vi "DFT.vi"(0 "dt":dbl=0.001, 1 "Input Y":dbl[](array[numeric]), 3 "Input X":dbl[](array[numeric]), 5 "df":dbl=1.0, 9 "fmin":dbl, 11 "fmax":dbl=500.0, 12 "Windowing":T3=enum."Sine", 13 "Autocorrelation before DFT":T1, 14 "Mean shifting":T2) -> (4 "Pwr out":dbl[](array[numeric]), 6 "fnyq.":dbl, 8 "Input to DFT":dbl[](graph), 10 "Actual fmin":dbl, 15 "Actual fmax":dbl)   [LabVIEW 2011]
uses:
  Windowing_list.ctl
  Mean_shift_list.ctl
  Autocorrelation_list.ctl
  <vilib>/Analysis/4window.llb/Cosine Tapered Window (DBL).vi
  <vilib>/Analysis/4window.llb/Triangle Window (DBL).vi
  <vilib>/Analysis/4window.llb/Exact Blackman Window (DBL).vi
  <vilib>/Analysis/4window.llb/Flat Top Window (DBL).vi
  <vilib>/Analysis/4window.llb/Hamming Window (DBL).vi
  <vilib>/Analysis/4window.llb/Hanning Window (DBL).vi
  <vilib>/Analysis/4window.llb/Blackman Window (DBL).vi
  <vilib>/Analysis/4window.llb/Blackman-Harris Window (DBL).vi
  <vilib>/Analysis/2dsp.llb/1D Auto Correlation (DBL).vi
  <vilib>/Analysis/NI_AALBase.lvlib
  <vilib>/Analysis/NI_AALPro.lvlib
panel:
  out "Variance Density Spectrum":cluster{"fmin":dbl, "df":dbl, dbl[]}(graph)
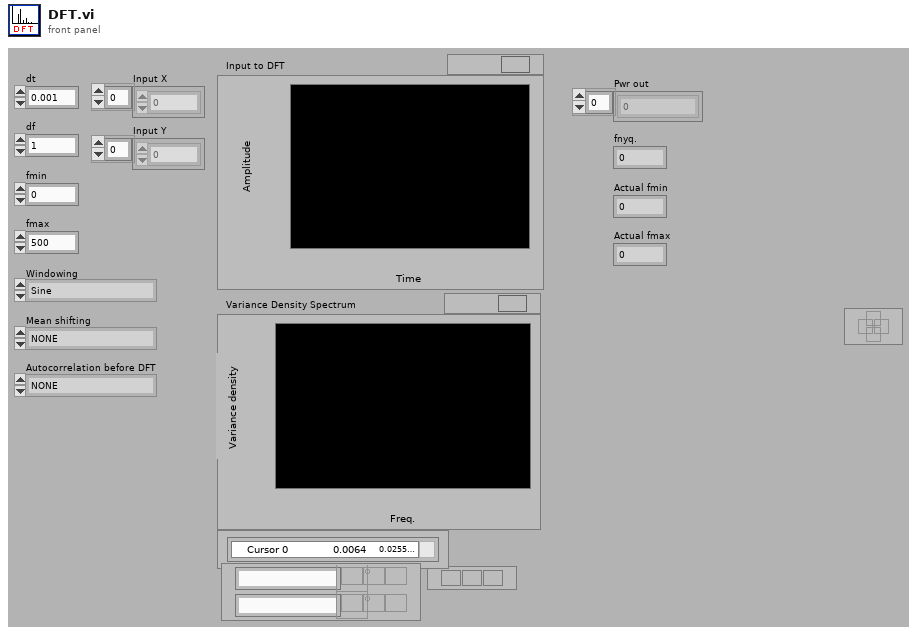
[diagram p1: front panel]
types:
  T1 = typedef "Autocorrelation_list.ctl" = enum16{"NONE", "Biased", "Un-biased"}
  T2 = typedef "Mean_shift_list.ctl" = enum16{"NONE", "Eliminate DC only", "Eliminate all linear trends"}
  T3 = typedef "Windowing_list.ctl" = enum16{"NONE", "Blackman", "Blackman Harris", "Cosine Taper", "Exact Blackman", "Flat Top", "Hamming", "Hanning", "Sine", "Triangle"}
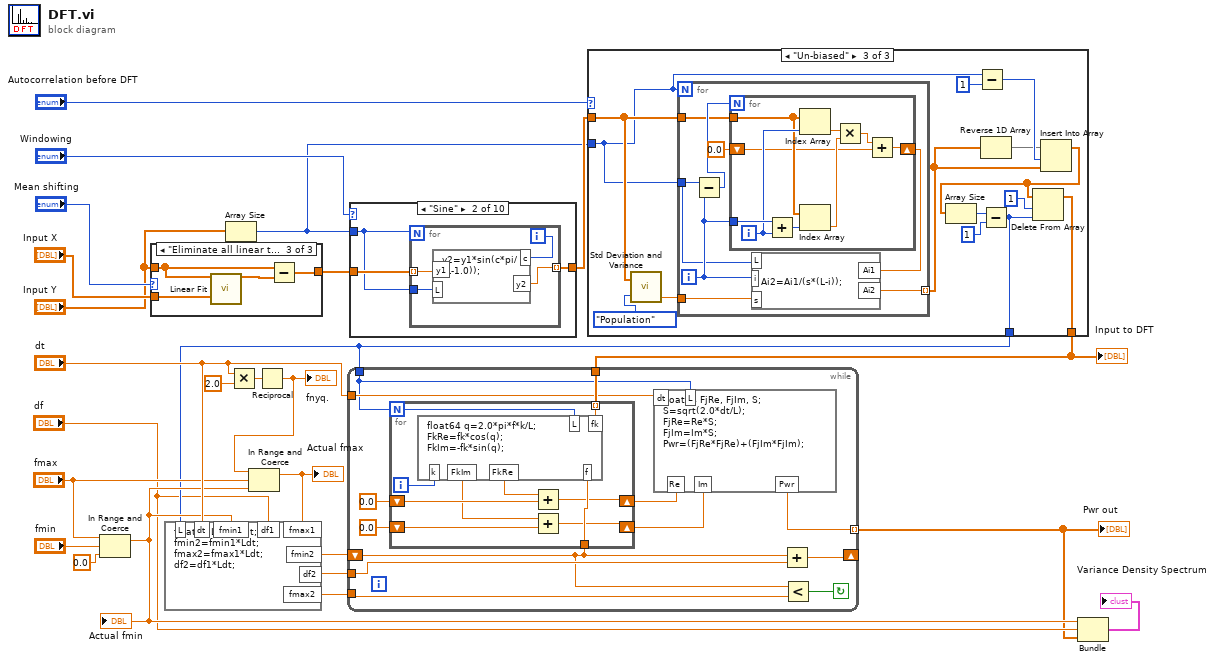
[diagram p0: block diagram]
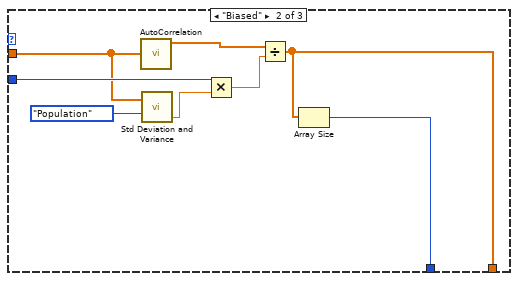
[diagram p3: hidden frame]
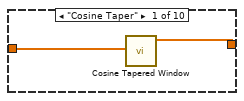
[diagram p4: hidden frame]
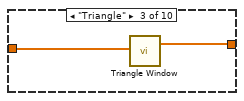
[diagram p5: hidden frame]
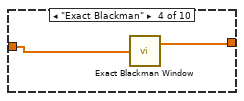
[diagram p6: hidden frame]
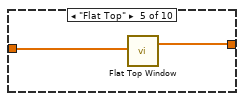
[diagram p7: hidden frame]
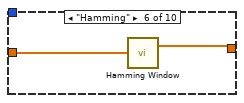
[diagram p8: hidden frame]
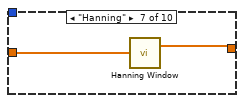
[diagram p9: hidden frame]
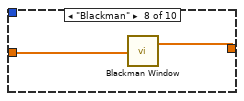
[diagram p10: hidden frame]
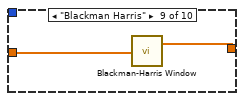
[diagram p11: hidden frame]
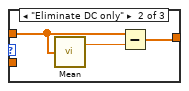
[diagram p14: hidden frame]
diagram:
  n1 = In Range and Coerce(upper limit="fmax", x="fmin", lower limit=0.0) -> (coerced(x)=w13:dbl)  [unwired: 1 out]
  "Actual fmin" <- w13
  n2 = case shown="\"Eliminate all linear trends\"" "Mean shifting" {
    tunnel: "Input Y" -> [w26 w27 w31]
    tunnel: [w26 w29 w30] -> w9
    tunnel: "Input X" -> [_ _ w33]
    frame "NONE" {
    }
    frame "Eliminate DC only" {
      n3 = call <vilib>:"Mean.vi"("X"=w27) -> ("mean"=w28:dbl)  [unwired: 1 out]
      n4 = Subtract(x=w27, y=w28) -> (x-y=w29:dbl[])
    }
    frame "Eliminate all linear trends" {
      n5 = call <vilib>:"Linear Fit.vi"("Y"=w31, "X"=w33) -> ("Best Linear Fit"=w32:dbl[])  [unwired: 9 in, 4 out]
      n6 = Subtract(x=w31, y=w32) -> (x-y=w30:dbl[])
    }
  }
  n7 = Array Size(array="Input Y") -> (size(s)=w4:i32)
  n8 = Multiply(x="dt", y=2.0) -> (x*y=w24:dbl)
  n9 = Reciprocal(x=w24) -> (1/x=w18:dbl)
  "fnyq." <- w18
  n10 = In Range and Coerce(upper limit=w18, x="fmax", lower limit=w13) -> (coerced(x)=w17:dbl)  [unwired: 1 out]
  "Actual fmax" <- w17
  n11 = case shown="\"Sine\"" "Windowing" {
    tunnel: w9 -> [w35 w37 w44 w46 w48 w50 w52 w54 w56 w57]
    tunnel: [w34 w38 w43 w45 w47 w49 w51 w53 w55 w57] -> w7
    tunnel: w4 -> [_ w36 _ _ _ _ _ _ _ _]
    frame "Cosine Taper" {
      n12 = call-poly <vilib>:"Cosine Tapered Window.vi"("X"=w35) -> ("Windowed X"=w34:dbl[])  [unwired: 9 in, 1 out]
    }
    frame "Sine" {
      n13 = for {
        N: w36 -> [_]
        tunnel: w37 -> [w42] mode=indexing
        tunnel: w36 -> [w41]
        tunnel: [w40] -> w38 mode=indexing
        i -> [w39]
        n14 = formula code="y2=y1*sin(c*pi/(L-1.0));"("y1"=w42, "L"=w41, "c"=w39) -> ("y2"=w40:dbl)
      }
    }
    frame "Triangle" {
      n15 = call-poly <vilib>:"Triangle Window.vi"("X"=w44) -> ("Windowed X"=w43:dbl[])  [unwired: 1 out]
    }
    frame "Exact Blackman" {
      n16 = call-poly <vilib>:"Exact Blackman Window.vi"("X"=w46) -> ("Windowed X"=w45:dbl[])  [unwired: 1 out]
    }
    frame "Flat Top" {
      n17 = call-poly <vilib>:"Flat Top Window.vi"("X"=w48) -> ("Windowed X"=w47:dbl[])  [unwired: 1 out]
    }
    frame "Hamming" {
      n18 = call-poly <vilib>:"Hamming Window.vi"("X"=w50) -> ("Windowed X"=w49:dbl[])  [unwired: 1 out]
    }
    frame "Hanning" {
      n19 = call-poly <vilib>:"Hanning Window.vi"("X"=w52) -> ("Windowed X"=w51:dbl[])  [unwired: 1 out]
    }
    frame "Blackman" {
      n20 = call-poly <vilib>:"Blackman Window.vi"("X"=w54) -> ("Windowed X"=w53:dbl[])  [unwired: 1 out]
    }
    frame "Blackman Harris" {
      n21 = call-poly <vilib>:"Blackman-Harris Window.vi"("X"=w56) -> ("Windowed X"=w55:dbl[])  [unwired: 1 out]
    }
    frame "NONE" {
    }
  }
  n22 = case shown="\"Un-biased\"" "Autocorrelation before DFT" {
    tunnel: w7 -> [w59 w61 w81]
    tunnel: [w58 w67 w68] -> w6
    tunnel: [w59 w65 w72] -> w1
    tunnel: w4 -> [w58 w64 w77]
    frame "NONE" {
    }
    frame "Biased" {
      n23 = call-poly <vilib>:"AutoCorrelation.vi"("X"=w61) -> ("Rxx"=w66:dbl[])  [unwired: 9 in, 1 out]
      n24 = call <vilib>:"Std Deviation and Variance.vi"("X"=w61, "Weighting (Sample)"=enum16{"Sample", "Population"}."Population") -> ("variance"=w62:dbl)  [unwired: 2 out]
      n25 = Multiply(x=w64, y=w62) -> (x*y=w63:dbl)
      n26 = Divide(x=w66, y=w63) -> (x/y=w65:dbl[])
      n27 = Array Size(array=w65) -> (size(s)=w67:i32)
    }
    frame "Un-biased" {
      n28 = call <vilib>:"Std Deviation and Variance.vi"("X"=w81, "Weighting (Sample)"=enum16{"Sample", "Population"}."Population") -> ("variance"=w79:dbl)  [unwired: 2 out]
      n29 = for {
        N: w77 -> [_]
        tunnel: w77 -> [w82]
        tunnel: w81 -> [w85]
        tunnel: w79 -> [w88]
        tunnel: [w86] -> w74 mode=indexing
        i -> [w87]
        n30 = Subtract(x=w82, y=w87) -> (x-y=w89:i32)
        n31 = for {
          N: w89 -> [_]
          tunnel: w87 -> [w96]
          tunnel: w85 -> [w93]
          shift-right: [w90] -> w83
          shift-left: 0.0 -> [w92]
          i -> [w95]
          n32 = Add(x=w96, y=w95) -> (x+y=w94:i32)
          n33 = Index Array(array=w93, index=w95) -> (element=w98:dbl)
          n34 = Index Array(array=w93, index=w94) -> (element=w97:dbl)
          n35 = Multiply(x=w98, y=w97) -> (x*y=w91:dbl)
          n36 = Add(x=w91, y=w92) -> (x+y=w90:dbl)
        }
        n37 = formula code="Ai2=Ai1/(s*(L-i));"("L"=w82, "i"=w87, "s"=w88, "Ai1"=w83) -> ("Ai2"=w86:dbl)
      }
      n38 = Subtract(x=w77, y=1) -> (x-y=w76:i32)
      n39 = Reverse 1D Array(array=w74) -> (reversed array=w75:dbl[])
      n40 = Insert Into Array(array=w75, index=w76, new element=w74) -> (w71:dbl[])
      n41 = Array Size(array=w71) -> (size(s)=w69:i32)
      n42 = Subtract(x=w69, y=1) -> (x-y=w68:i32)
      n43 = Delete From Array(array=w71, length=1, index=w68) -> (array with subset deleted=w72:dbl[])  [unwired: 1 out]
    }
  }
  "Input to DFT" <- w1
  n44 = formula code="float64 Ldt=L*dt;\nfmin2=fmin1*Ldt;\nfmax2=fmax1*Ldt;\ndf2=df1*Ldt;"("L"=w6, "dt"="dt", "fmin1"=w13, "fmax1"=w17, "df1"="df") -> ("fmin2"=w21:dbl, "fmax2"=w22:dbl, "df2"=w20:dbl)
  n45 = while {
    tunnel: w6 -> [w107]
    tunnel: w20 -> [w101]
    tunnel: "dt" -> [w108]
    tunnel: w1 -> [w109]
    tunnel: [w99] -> w2 mode=indexing
    shift-right: [w104] -> _
    shift-left: w21 -> [w100]
    tunnel: w22 -> [w102]
    stop <- w103 continue-if-true
    n46 = for {
      N: w107 -> [w121]
      shift-right: [w117] -> w106
      shift-left: 0.0 -> [w115]
      tunnel: w100 -> [w120]
      shift-right: [w118] -> w105
      shift-left: 0.0 -> [w116]
      tunnel: w109 -> [w112] mode=indexing
      i -> [w119]
      n47 = formula code="float64 q=2.0*pi*f*k/L;\nFkRe=fk*cos(q);\nFkIm=-fk*sin(q);"("fk"=w112, "k"=w119, "L"=w121, "f"=w120) -> ("FkRe"=w114:dbl, "FkIm"=w113:dbl)
      n48 = Add(x=w114, y=w115) -> (x+y=w117:dbl)
      n49 = Add(x=w113, y=w116) -> (x+y=w118:dbl)
    }
    n50 = formula code="float64 FjRe, FjIm, S;\nS=sqrt(2.0*dt/L);\nFjRe=Re*S;\nFjIm=Im*S;\nPwr=(FjRe*FjRe)+(FjIm*FjIm);"("dt"=w108, "L"=w107, "Re"=w106, "Im"=w105) -> ("Pwr"=w99:dbl)
    n51 = Add(x=w100, y=w101) -> (x+y=w104:dbl)
    n52 = Less?(x=w100, y=w102) -> (x < y?=w103:bool)
  }
  "Pwr out" <- w2
  n53 = Bundle("fmax"=w13, "df"="df", w2) -> (→"Variance Density Spectrum":cluster{"fmax":dbl, "df":dbl, dbl[]})  [unwired: 1 in]
